vi "Write Desired Temperature.vi"(10 "Desired Temperature":dbl=75.0, 11 "Cooler in":refnum<class "Cooler.lvclass">) -> (3 "Cooler out":refnum<class "Cooler.lvclass">)   [LabVIEW 2018, in "Cooler.lvlib" / "Cooler.lvclass"]
doc: "Writes the temperature that the system is aiming to maintain."
uses:
  Cooler.lvclass
  e:/builds/penguin/labview/branches/2018/dev/dist/ProjectTemplates/Source/Core/Feedback Evaporative Cooler/Level Controller/Level Controller/Level Controller.lvclass
  Level Controller/Level Controller/Deadband.ctl
  Level Controller/Level Controller/Level Controller.lvclass
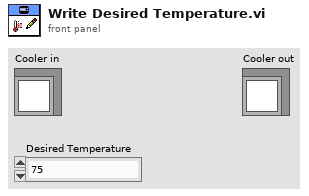
[diagram p1: front panel]
types:
  T1 = typedef "Level Controller.lvlib/Level Controller.lvclass/Deadband.ctl" = cluster{"Low":dbl, "High":dbl}
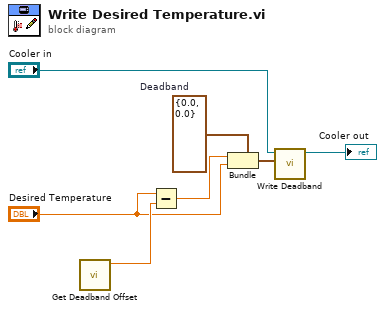
[diagram p0: block diagram]
diagram:
  w1 = T1 {"Low"=0.0, "High"=0.0}  # Deadband
  n1 = call "Get Deadband Offset.vi"() -> ("deadband offset"=w7:dbl)  [unwired: 11 in]
  n2 = Subtract(x="Desired Temperature", y=w7) -> (x-y=w6:dbl)
  n3 = Bundle(cluster=w1, "Low"=w6, "High"="Desired Temperature") -> (w2:T1)
  n4 = call "Write Deadband.vi"("Deadband"=w2, "Level Controller in"="Cooler in") -> ("Level Controller out"=→"Cooler out":refnum<class "Cooler.lvclass">)  [unwired: 8 in, 1 out]
